vi "Soft_Robot_Model_ffwd.vi"() -> ()   [LabVIEW 2015]
uses:
  <vilib>/addons/Control Design/_Stochastic Systems/Stochastic Systems.llb/Stochastic Systems SubVIs/cd_Stochastic State-Space Model.ctl
  <vilib>/addons/Control Design/_Model Construction/Model Typedefs.llb/CD State Space Model (MIMO).ctl
  <vilib>/addons/Control Design/_Model Construction/Model Typedefs.llb/CD General Elements.ctl
  <vilib>/Analysis/Matrix/Datatypes/RealMatrix.ctl
  <vilib>/addons/Control Design/_Stochastic Systems/Stochastic Systems.llb/CD CtoD Stochastic Model.ctl
  <vilib>/Analysis/7linalg.llb/Eigenvalue and Vectors Output Option.ctl
  <vilib>/Platform/TimedLoop/XDataNode/timing_clust.ctl
  <vilib>/Platform/TimedLoop/XDataNode/nitl_modes.ctl
  <vilib>/Platform/TimedLoop/XDataNode/wakeup.ctl
  <vilib>/Simulation/Scripting/Companion Diagram/SimConfigNode/SimParams.ctl
  <vilib>/Simulation/Scripting/Companion Diagram/SimConfigNode/_simSolvers.ctl
  <vilib>/Simulation/Implementation/Shared/SIMSCR Execution Mode.ctl
  <vilib>/Simulation/Param Hierarchy/Typedefs/SIMPH Param Control Actions.ctl
  <vilib>/Simulation/Implementation/Shared/NILVSim_ParamChanged.vi
  <vilib>/Simulation/Implementation/Shared/NILVSim_FinishedLate.vi
  <vilib>/Simulation/Implementation/Shared/NILVSIM_BeginStep.vi
  <vilib>/Simulation/SignalArithmetic/Implementation/NILVSim Gain.llb/SIM Gain (scalar).vi
  <vilib>/Simulation/Implementation/Shared/NILVSim_Manager.vi
  <vilib>/Utility/error.llb/Clear Errors.vi
  <vilib>/Simulation/Implementation/Shared/NILVSim_FinalizeModel.vi
  <vilib>/addons/Control Design/_Stochastic Systems/Stochastic Systems.llb/CD Construct Stochastic Model (Numeric).vi
  <vilib>/Analysis/7linalg.llb/Create Special Real Matrix.vi
  <vilib>/addons/Control Design/_Stochastic Systems/Stochastic Systems.llb/CD Construct Noise Model (Numeric).vi
  <vilib>/Analysis/7linalg.llb/Real Eigenvalues and Vectors.vi
  <vilib>/addons/Control Design/_State Feedback Control/State Feedback Control.llb/State Feedback Control SubVis/cd_Linear Quadratic Regulator.vi
  <vilib>/FPGAPlugInAG/myRIO-1900/niLvFpga_Open_myRIO-1900.vi
  <vilib>/rvi/interface/common/dynamic/niFpgaDynamicAddResources.vi
  <vilib>/Utility/error.llb/Error Cluster From Error Code.vi
  <vilib>/rvi/errors/niLvFpgaAdjustHostInterfaceError.vi
  <vilib>/FPGAPlugInAG/Dynamic/niLvFpga_Close_Dynamic.vi
  <vilib>/Simulation/Implementation/Shared/SIM Unbundle Sim Info.vi
  <vilib>/Simulation/Implementation/Shared/SIMSH Read Queue.vi
  <vilib>/Simulation/Implementation/Shared/NILVSim_Initialize.vi
  <vilib>/Utility/file.llb/Write Delimited Spreadsheet.vi
  <vilib>/Utility/file.llb/Write Delimited Spreadsheet (DBL).vi
  <vilib>/Simulation/Utility/Implementation/NILVSim Get Time and IsAcceptedStep.vi
  <vilib>/Simulation/Estimation/Implementation/NILVSim Discrete Kalman Filter.llb/SIM Disc KF Pred and Corr with Pred Gain with Checking Indirect Distributor Sim.vi
  <vilib>/addons/Control Design/_Implementation/CD State Feedback Controller.vi
  <vilib>/addons/Control Design/_Implementation/CD State Feedback Controller (Multiple Outputs).vi
  <vilib>/Simulation/Estimation/Implementation/NILVSim Discrete Kalman Filter.llb/SIM Disc KF Pred and Corr with Pred Gain with Checking Indirect Collector Sim.vi
  <vilib>/Simulation/Implementation/Shared/NILVSim_GetModelError.vi
  <vilib>/Simulation/Implementation/Shared/SIM Bundle Sim Info.vi
  <vilib>/Platform/TimedLoop/XDataNode/XDataNode.xnode
  <vilib>/rvi/interface/nirviOpenFPGA/nirviOpenFPGA.xnode
  FPGA Bitfiles/ACC20115_FPGATarget_CurrentControlle_W-6n2rsGK8k.lvbitx
  Misc/Current Controller.vi
  <vilib>/rvi/interface/nirviReadWriteControl/nirviReadWriteControl.xnode
  <vilib>/rvi/interface/nirviCloseFPGA/nirviCloseFPGA.xnode
  <vilib>/Simulation/Scripting/Companion Diagram/SimConfigNode/SimDog.xnode
  <vilib>/Simulation/Implementation/XNodeFramework/SimXNode/SimX.xnode
  <vilib>/addons/Control Design/_State Feedback Control/NI_CD_State Feedback Control.lvlib
  <vilib>/Analysis/NI_AALPro.lvlib
  <vilib>/Platform/TimedLoop/XDataNode/XDNodeRunTimeDep.lvlib
  <vilib>/rvi/interface/Simulation/niFpgaSimulationCallBeginRW.vi
  <vilib>/addons/Control Design/_Stochastic Systems/NI_CD_Stochastic Systems.lvlib
  <vilib>/addons/Control Design/_State-Space Analysis/NI_CD_State-Space Analysis.lvlib
  NiFpgaLv.dll
  <vilib>/addons/Control Design/_Implementation/NI_CD_Implementation.lvlib
  <vilib>/Simulation/Estimation/Implementation/NILVSim Discrete Kalman Filter.llb/SIM Disc KF Pred and Corr with Pred Gain with Checking Indirect Sim.vi
  <vilib>/Simulation/Implementation/Shared/NI_SIM_Implementation.lvlib
  <vilib>/addons/Control Design/_Model Construction/NI_LinSys_Model Typedefs.lvlib
  <vilib>/Analysis/Matrix/NI_Matrix.lvlib
panel:
  out "Kffwd":dbl
  in  "Current (mA)":i32
  in  "Tab Control":enum32{"Outputs", "SS Outs", "Inputs"}(tab)
  out "Valve Current (mA)":dbl(graph)
  out "Kinect Fusion":dbl(graph)
  out "Plant Output and KF estimation":dbl[][](graph)=[[694.135, 693.2125685090368]]
  in  "Stop":bool
  out "Control Action":dbl
  out "Controllable?":bool
  out "Stable?":bool
  out "Detectable?":bool
  out "Observable?":bool
  out "FPGA Overflow?":bool
  in  "SP (mm)":dbl(knob)=687.2508300641372 scale=670.0..695.0
  out "Local Kalman Filters & Central Site Fusion":dbl[][](graph)
  in  "K_ffd":dbl(knob) scale=-35.0..10.0
  out "Stochastic SS Model":T1={"Sampling Time (s)"=0.0, "G"=[], "B"=[[-1.71e-07], [6.47e-07]], "A"=[], "C"=[], "D"=[], "H"=[]} {"H" format="%#.2g"; "D" format="%#.2g"; "C" format="%#.2g"; "A" format="%#.2g"; "B" format="%#.2g"; "G" format="%#.2g"; "Sampling Time (s)" format="%.2f"}
  out "Deterministic SS Model":T2={"properties"={"Model name"="", "Input names"=[], "Output names"=[], "Input Delays"=[], "Output Delays"=[], "Sampling Time"=0.0, "Notes"=""}, "A"=[], "B"=[[-1.706e-07], [6.469e-07]], "C"=[], "D"=[], "StateNames"=[], "Transport Delay"=[]} {"Transport Delay" format="%.2f"; "D" format="%#.2g"; "C" format="%#.2g"; "B" format="%#.2g"; "A" format="%#.2g"; "properties"."Sampling Time" format="%#.6p"; "properties"."Output Delays" format="%.4f"; "properties"."Input Delays" format="%.4f"}
  out "DAC Loop Error":errorcluster
  out "LQR Error":errorcluster
  out "FPGA Loop Error":errorcluster
  out "KF Model Error":errorcluster
  out "UDP Loop Error":errorcluster
  out "LQR R Matrix":T4
  out "LQR Q Matrix":T4
  out "Optimal LQR Gains":dbl[][](array[numeric])
  out "LQR Eigenvalues":cdb[](array[numeric]) format="%.5f"
  out "LQR Q Eig Vals":cdb[](array[numeric])
  out "LQR R Eig Val":cdb[](array[numeric])
  out "KF Gain M(k)":dbl[][](array[numeric]) format="%#.6g"
  out "KF Predictor Gain L(k)":dbl[][](array[numeric])=[[1.0]] format="%#.6g"
  out "P(k+1|k)":dbl[][](array[numeric])
  out "P(k|k)":dbl[][](array[numeric])
  out "KF R Matrix":T4
  out "KF Q Matrix":T4
  out "Error":errorcluster
  in  "A":dbl[][](array[numeric])=[[-0.275, -0.05848], [0.3155, 0.05955]] format="%#.5g"
  in  "B":dbl[][](array[numeric])=[[-0.0001629], [8.009e-05]] format="%#.5g"
  in  "C":dbl[][](array[numeric])=[[0.742, 2.316]] format="%#.5g"
  in  "G":dbl[][](array[numeric])=[[0.7998], [2.296]] format="%#.2g"
  in  "xhat(0|-1)":dbl[](array[numeric])=[687.0, 687.0]
  in  "P(0|-1)":dbl[][](array[numeric])=[[1.0, 0.0], [0.0, 1.0]]
  in  "KF R":dbl[](array[knob]) scale=0.0..100.0
  in  "KF Q":dbl[](array[knob]) scale=0.0..100.0
  in  "LQR R":dbl[](array[knob]) scale=0.001..0.1
  in  "LQR Matrix (Q)":dbl[](array[knob]) scale=0.0..2.0
  in  "yfusion":path
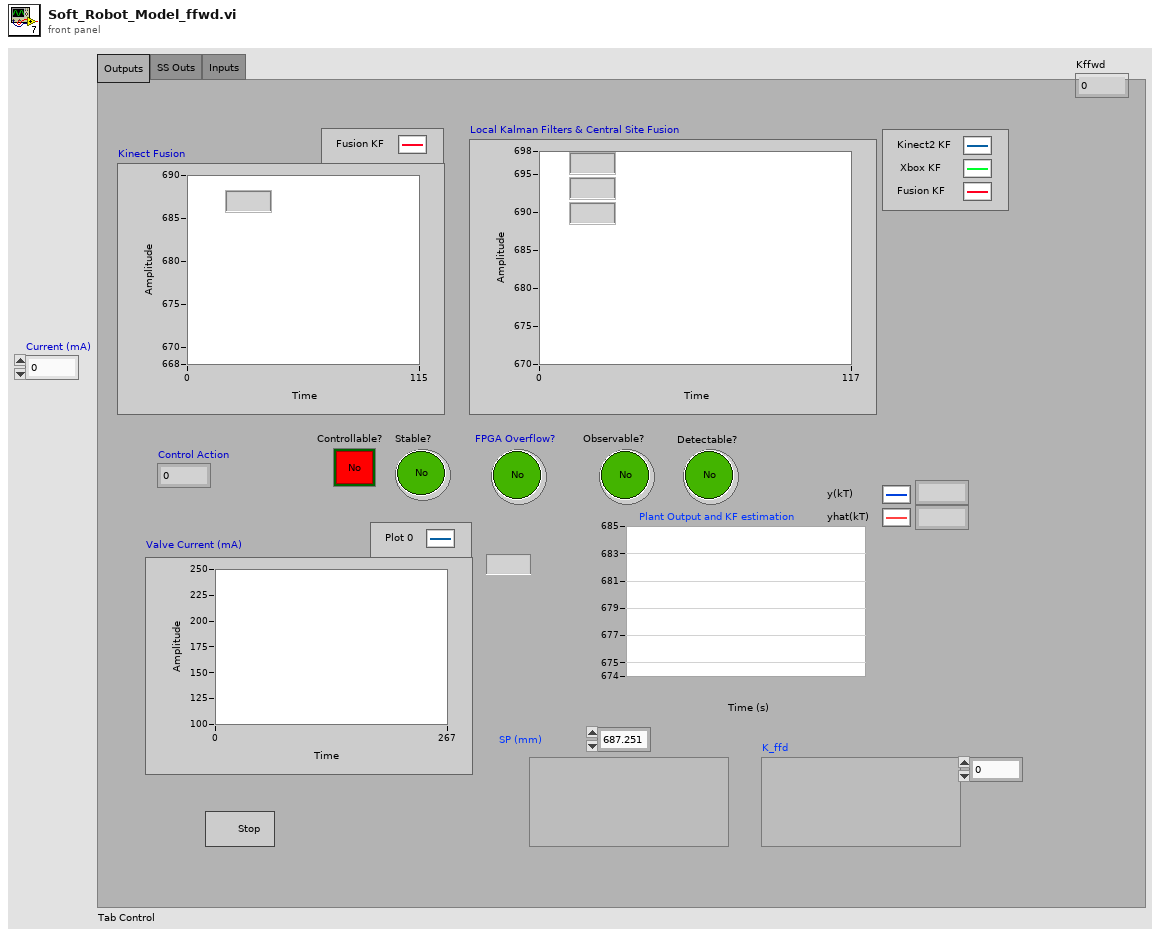
[diagram p1: front panel]
types:
  T1 = typedef "NI_CD_Stochastic Systems.lvlib/cd_Stochastic State-Space Model.ctl" = cluster{"Sampling Time (s)":dbl, "G":dbl[][], "B":dbl[][], "A":dbl[][], "C":dbl[][], "D":dbl[][], "H":dbl[][]}
  T2 = typedef "NI_LinSys_Model Typedefs.lvlib/CD State Space Model (MIMO).ctl" = cluster{"properties":T3, "A":dbl[][], "B":dbl[][], "C":dbl[][], "D":dbl[][], "StateNames":string[], "Transport Delay":dbl[][]}
  T3 = typedef "NI_LinSys_Model Typedefs.lvlib/CD General Elements.ctl" = cluster{"Model name":string, "Input names":string[], "Output names":string[], "Input Delays":dbl[], "Output Delays":dbl[], "Sampling Time":dbl, "Notes":string}
  T4 = typedef "NI_Matrix.lvlib/RealMatrix.ctl" = dbl[][]
  T5 = typedef "NI_AALPro.lvlib/Eigenvalue and Vectors Output Option.ctl" = i32
  T6 = enum32{"Identity", "Diagonal", "Toepliz", "Vandermonde", "Companion"}
  T7 = typedef "NI_CD_Stochastic Systems.lvlib/CD CtoD Stochastic Model.ctl" = enum16{"Truncation of Taylor Series", "Numerical Integration"}
  T8 = enum16{"state weighting", "output weighting, Dim Q = Ny", "output weighting, Dim Q = Nx"}
  T9 = typedef "NI_CD_Stochastic Systems.lvlib/cd_Second-Order Statistics Noise Model.ctl" = cluster{"Q":dbl[][], "E{w}":dbl[], "E{v}":dbl[], "R":dbl[][], "N":dbl[][]}
  T10 = typedef "XDNodeRunTimeDep.lvlib/timing_clust.ctl" = cluster{"Expected End [f-1]":u64, "Actual End [f-1]":u64, "Finished Late? [f-1]":bool, "Expected End [i-1]":u64, "Actual End [i-1]":u64, "Finished Late? [i-1]":bool, "Expected Start [i]":u64, "Actual Start [i]":u64, "Expected Start [f]":u64, "Actual Start [f]":u64, "Source Name":string, "Structure Name":string, "Period":i64, "Deadline":i64, "Offset":i64, "Start":i64, "Priority":i32, "Timeout":i32, "Mode":T11, "Wakeup Reason":T12, "Error":errorcluster, "Source Type":string, "Secondary Source Type":string, "Global End Time":u64, "Global Start Time":u64, "Frame Duration":u64, "Iteration Duration":u64, "Assigned CPU":i32, "I/O Scan Engine Mode":u32}
  T11 = typedef "XDNodeRunTimeDep.lvlib/nitl_modes.ctl" = enum32{"No Change", "Process missed periods, maintain original phase", "Discard missed periods, maintain original phase", "Process missed periods, ignore original phase", "Discard missed periods, ignore original phase"}
  T12 = typedef "XDNodeRunTimeDep.lvlib/wakeup.ctl" = enum32{"Normal", "Aborted", "Asynchronous wakeup", "Timing source error", "Timed loop error", "Timeout"}
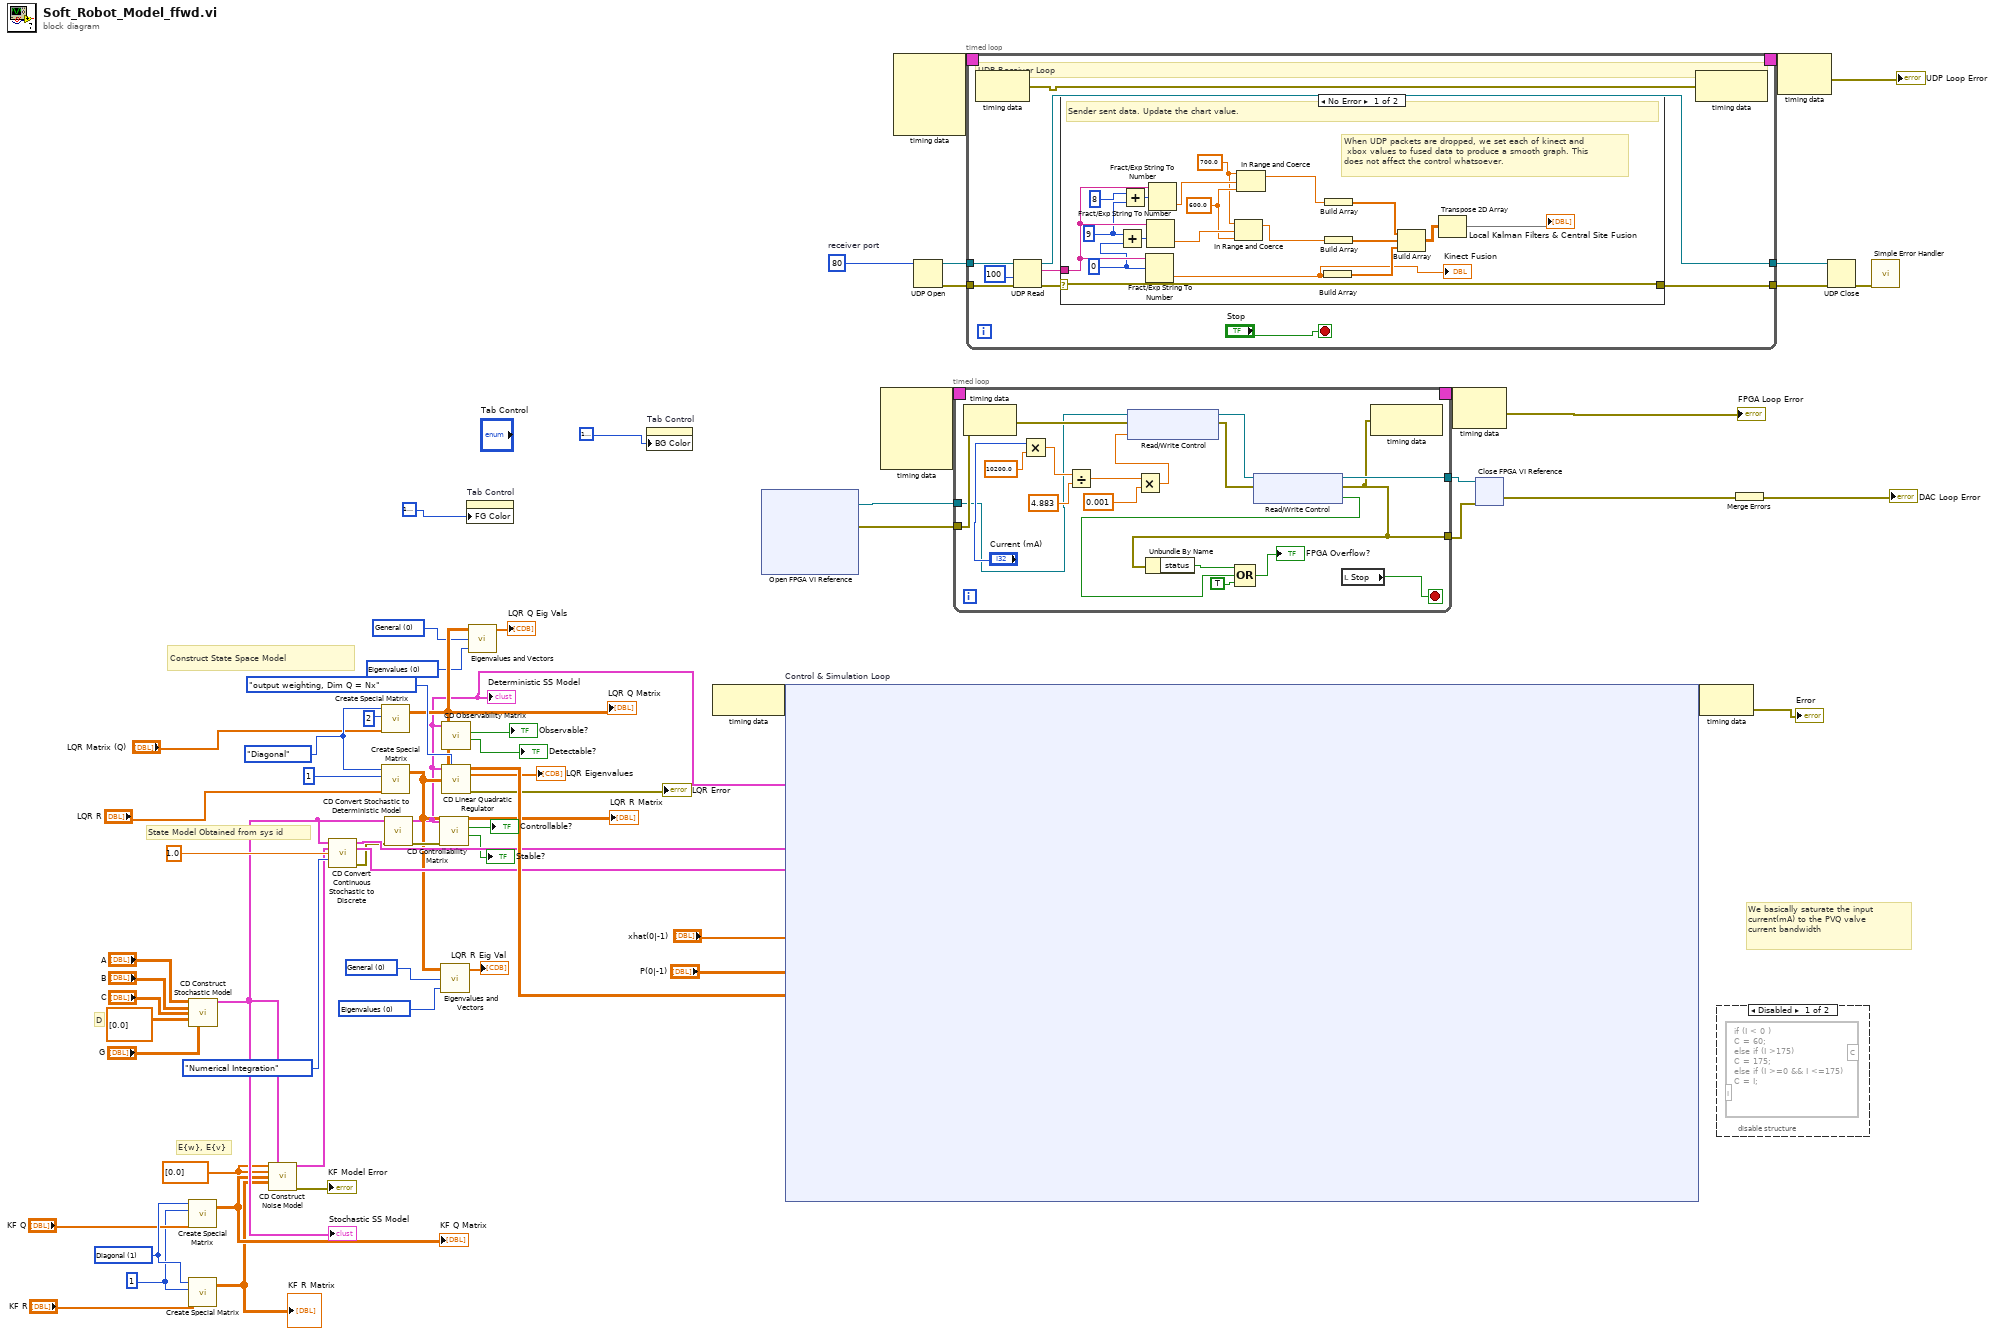
[diagram p0: block diagram]
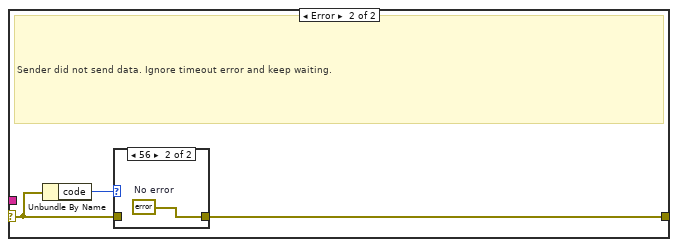
[diagram p3: hidden frame]
diagram:
  w18 = T5 0 items=["Eigenvalues", "Eigenvalues & Vectors"] ("output option")
  w19 = 0 items=["General", "Symmetric"] ("matrix type")
  w21 = T5 0 items=["Eigenvalues", "Eigenvalues & Vectors"] ("output option")
  w22 = 0 items=["General", "Symmetric"] ("matrix type")
  w26 = T6."Diagonal" ("matrix type")
  w27 = 1 ("KF Q/R Size")
  w31 = dbl[] [0.0] ("E{w}")
  w32 = 1 items=["Identity", "Diagonal", "Toeplitz", "Vandermonde", "Companion", "Hankel", "Hadamard", "Wilkinson", "Hilbert", "Inverse Hilbert", "Rosser", "Pascal"] ("matrix type")
  w56 = u16 80  # receiver port
  # "We basically saturate the input current(mA) to the PVQ valve current bandwidth"
  # "E{w}, E{v}"
  # "D"
  # "State Model Obtained from sys id"
  # "Construct State Space Model"
  n1 = call-poly <vilib>:"Create Special Matrix.vi"("matrix type"=w32, "matrix size"=w27, "Input Vector1"="KF Q") -> ("Special Matrix"=w34:T4)  [unwired: 2 in, 1 out]
  "KF Q Matrix" <- w34
  n2 = call-poly <vilib>:"Create Special Matrix.vi"("matrix type"=w32, "matrix size"=w27, "Input Vector1"="KF R") -> ("Special Matrix"=w33:T4)  [unwired: 2 in, 1 out]
  "KF R Matrix" <- w33
  n3 = call-poly <vilib>:"CD Construct Stochastic Model.vi"("A"="A", "B"="B", "C"="C", "D"=dbl[][] [[0.0]], "G"="G") -> ("Stochastic State-Space Model"=w40:T1)  [unwired: 3 in, 7 out]
  "Stochastic SS Model" <- w40
  n4 = call-poly <vilib>:"CD Construct Noise Model.vi"("E{w}"=w31, "Stochastic State-Space Model"=w40, "E{v}"=w31, "Q"=w34, "R"=w33) -> ("Second-Order Statistics Noise Model out"=w41:T9, "error out"=→"KF Model Error":errorcluster)  [unwired: 2 in, 7 out]
  n5 = call <vilib>:"CD Convert Continuous Stochastic to Discrete.vi"("Continuous Stochastic\nState-Space Model"=w40, "Continuous Second-Order\nStatistics Noise Model"=w41, "Sampling Time (s)"=1.0, "Method"=CD_CtoD_Stochastic_Model."Numerical Integration") -> ("Discrete Stochastic\nState-Space Model"=w50:T1, "Discrete Second-Order\nStatistics Noise Model"=w51:T9, "error out"=w39:errorcluster)  [unwired: 1 in, 8 out]
  n6 = call-poly <vilib>:"Create Special Matrix.vi"("matrix type"=w26, "matrix size"=2, "Input Vector1"="LQR Matrix (Q)") -> ("Special Matrix"=w23:T4)  [unwired: 2 in, 1 out]
  "LQR Q Matrix" <- w23
  n7 = call-poly <vilib>:"Create Special Matrix.vi"("matrix type"=w26, "matrix size"=1, "Input Vector1"="LQR R") -> ("Special Matrix"=w16:T4)  [unwired: 2 in, 1 out]
  "LQR R Matrix" <- w16
  n8 = call <vilib>:"CD Convert Stochastic to Deterministic Model.vi"("Stochastic State-Space Model"=w40, "error in (no error)"=w39) -> ("Deterministic State-Space Model"=w1:T2, "error out"=w38:errorcluster)  [unwired: 12 in]
  "Deterministic SS Model" <- w1
  n9 = call <vilib>:"CD Controllability Matrix.vi"("error in (no error)"=w38, "State-Space Model"=w1) -> ("Is Stabilizable?"=→"Stable?":bool, "Is Controllable?"=→"Controllable?":bool)  [unwired: 6 in, 2 out]
  n10 = call-poly <vilib>:"Eigenvalues and Vectors.vi"("output option"=w18, "matrix type"=w19, "Input Matrix"=w16) -> ("Eigenvalues"=→"LQR R Eig Val":cdb[])  [unwired: 2 out]
  n11 = call <vilib>:"CD Observability Matrix.vi"("State-Space Model"=w1) -> ("Is Detectable?"=→"Detectable?":bool, "Is Observable?"=→"Observable?":bool)  [unwired: 7 in, 2 out]
  n12 = call-poly <vilib>:"CD Linear Quadratic Regulator.vi"("State-Space Model"=w1, "Weighting Type"=T8."output weighting, Dim Q = Nx", "Q"=w23, "R"=w16) -> ("Optimal Gain (K)"=w52:dbl[][], "Eigenvalues"=→"LQR Eigenvalues":cdb[], "error out"=→"LQR Error":errorcluster)  [unwired: 8 in, 1 out]
  n13 = property on="Tab Control" class="TabCtl (strict)"("FG Color"=u32 16777226) -> ()  [unwired: 2 in, 2 out]
  n14 = call-poly <vilib>:"Eigenvalues and Vectors.vi"("output option"=w21, "matrix type"=w22, "Input Matrix"=w23) -> ("Eigenvalues"=→"LQR Q Eig Vals":cdb[])  [unwired: 2 out]
  n15 = property on="Tab Control" class="TabCtl (strict)"("BG Color"=u32 16777226) -> ()  [unwired: 2 in, 2 out]
  n16 = node-c288() -> (w4:variant)  [unwired: 1 in]
  n17 = xnode "Open FPGA VI Reference"() -> ("FPGA VI Reference Out"=w9:refnum<k20>, "error out"=w8:errorcluster)  [unwired: 2 in]
  n18 = node-c254 "Control & Simulation Loop"(w4, w51, "xhat(0|-1)", "P(0|-1)", w50, w1, w52) -> (w3:variant)
  n19 = node-c288() -> (w66:T10)  [unwired: 4 in]
  n20 = node-c288() -> (w55:T10)  [unwired: 4 in]
  n21 = UDP Open(11:w56) -> (port=w57:refnum<k16>, 0:w58:errorcluster)  [unwired: 4 in, 1 out]
  n22 = timed-loop {
    tunnel: w8 -> [w73]
    tunnel: [w72] -> w64
    tunnel: [w81] -> w68
    timing: w66 -> [_]
    timing-out: [_] -> w65
    tunnel: w9 -> [w71]
    stop <- w70 stop-if-true
    n23 = node-c288() -> ()  [unwired: 1 in, 1 out]
    n24 = Multiply(x="Current (mA)", y=10200.0) -> (x*y=w76:dbl)
    n25 = Divide(x=w76, y=4.883) -> (x/y=w79:dbl)
    n26 = Multiply(x=w79, y=0.001) -> (x*y=w75:dbl)
    n27 = xnode "Read/Write Control"("FPGA VI Reference In"=w71, "error in"=w73, "DAC Inlet Valve"=w75) -> ("FPGA VI Reference Out"=w86:refnum<k20>, "error out"=w85:errorcluster)
    n28 = xnode "Read/Write Control"("FPGA VI Reference In"=w86, "error in"=w85) -> ("FPGA VI Reference Out"=w81:refnum<k20>, "error out"=w72:errorcluster, "Inlet Overflow?"=w82:bool)
    n29 = Unbundle By Name(w72) -> ("status"=w83:bool)
    n30 = Compound Arithmetic op=OR(w83, w82, TRUE ("value")) -> (→"FPGA Overflow?":bool)
    n31 = local read "Stop"() -> (w70:bool)
    n32 = node-c288(w72) -> ()  [unwired: 1 out]
  }
  n33 = timed-loop {
    tunnel: w57 -> [w99]
    tunnel: [w93] -> w61
    tunnel: w58 -> [w98]
    tunnel: [w94] -> w59
    timing: w55 -> [_]
    timing-out: [_] -> w54
    stop <- "Stop" stop-if-true
    # "UDP Receiver Loop"
    n34 = node-c288() -> (w91:errorcluster)  [unwired: 1 in]
    n35 = UDP Read(connection ID=w99, timeout ms (25000)=100, 8:w98) -> (data out=w96:string, error out=w95:errorcluster, 3:w93:refnum<k16>)  [unwired: 3 out]
    n36 = case shown="No Error" w95 {
      selector: w95 -> [w123 w125]
      tunnel: w96 -> [w122 _]
      tunnel: [w123 w124] -> w94
      frame No Error {
        w107 = 600.0 ("lower limit")
        w106 = 700.0 ("upper limit")
        w118 = 9 ("x")
        w120 = 0 ("offset")
        # "When UDP packets are dropped, we set each of kinect and\n xbox values to fused data to produce a smooth graph. This does not affect the control whatsoever."
        # "Sender sent data. Update the chart value."
        n37 = Add(x=w118, y=w120) -> (x+y=w121:i32)
        n38 = Add(x=8, y=w118) -> (x+y=w119:i32)
        n39 = Fract/Exp String To Number(string=w122, offset=w120) -> (number=w112:dbl)  [unwired: 2 in, 1 out]
        "Kinect Fusion" <- w112
        n40 = Fract/Exp String To Number(string=w122, offset=w121) -> (number=w108:dbl)  [unwired: 2 in, 1 out]
        n41 = Fract/Exp String To Number(string=w122, offset=w119) -> (number=w111:dbl)  [unwired: 2 in, 1 out]
        n42 = In Range and Coerce(upper limit=w106, x=w108, lower limit=w107) -> (coerced(x)=w109:dbl)  [unwired: 1 out]
        n43 = In Range and Coerce(upper limit=w106, x=w111, lower limit=w107) -> (coerced(x)=w110:dbl)  [unwired: 1 out]
        n44 = Build Array(w112) -> (w115:dbl[])
        n45 = Build Array(w110) -> (w114:dbl[])
        n46 = Build Array(w109) -> (w116:dbl[])
        n47 = Build Array(w114, w116, w115) -> (w113:dbl[][])
        n48 = Transpose 2D Array(2D array=w113) -> (transposed array=→"Local Kalman Filters & Central Site Fusion":dbl[][])
      }
      frame Error {
        # "Sender did not send data. Ignore timeout error and keep waiting."
        n49 = Unbundle By Name(w125) -> ("code"=w126:i32)
        n50 = case shown="56" w126 {
          tunnel: w125 -> [w127 _]
          tunnel: [w127 w128] -> w124
          frame Default {
          }
          frame 56 {
            w128 = errorcluster {"status"=FALSE, "code"=0, "source"=""}  # No error
          }
        }
      }
    }
    n51 = node-c288(w91) -> ()  [unwired: 1 out]
  }
  n52 = node-c288(w65) -> (→"FPGA Loop Error":errorcluster)
  n53 = xnode "Close FPGA VI Reference"("FPGA VI Reference In"=w68, "error in"=w64) -> ("error out"=w63:errorcluster)
  n54 = node-c288(w3) -> (→"Error":errorcluster)
  n55 = disable-structure shown="Disabled" {
    frame Disabled {
      n56 = formula code="if (I < 0 )\nC = 60;\nelse if (I >175)\nC = 175;\nelse if (I >=0 && I <=175)\nC = I;"() -> ()  [unwired: 1 in, 1 out]
    }
    frame Enabled {
    }
  }
  n57 = Merge Errors(w63) -> (→"DAC Loop Error":errorcluster)
  n58 = node-c288(w54) -> (→"UDP Loop Error":errorcluster)
  n59 = UDP Close(connection ID=w61, 8:w59) -> (error out=w60:errorcluster)  [unwired: 1 out]
  n60 = call <vilib>:"Simple Error Handler.vi"("error in (no error)"=w60) -> ()  [unwired: 1 in, 8 out]
